vi "Periodic Tasks.vi"(8 "error in (no error)":errorcluster) -> ()   [LabVIEW 2012]
doc: "This VI runs in parallel to other tasks. It can contain as many user-defined periodic loops as you need. These can carry out PID or other sorts of timed response."
uses:
  <vilib>/Rock Robotics/SystemInterfaces/Utilities/FPGA_UtilitiesLED Source.ctl
  <vilib>/Rock Robotics/SystemInterfaces/Utilities/FPGA_UtilitiesLED State.ctl
  <vilib>/Rock Robotics/WPI/Solenoid/WPI_SolenoidValue.ctl
  <vilib>/Rock Robotics/WPI/Compressor/WPI_CompressorGetSetRefNum.vi
  System Set Points and States.vi
  <vilib>/Rock Robotics/WPI/Solenoid/WPI_SolenoidSetEnum.vi
  Robot Global Data.vi
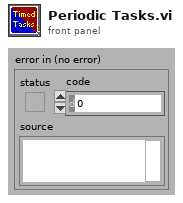
[diagram p1: front panel]
types:
  T1 = typedef "FPGA_UtilitiesLED State.ctl" = enum16{"Off", "On", "Toggle"}
  T2 = typedef "FPGA_UtilitiesLED Source.ctl" = enum16{"User LED", "FPGA LED"}
  T3 = typedef "WPI_SolenoidValue.ctl" = enum16{"Off", "On", "Forward", "Reverse"}
  T4 = typedef "WPI_SolenoidDevRef.ctl" = cluster{"DevStatus":errorcluster, "Solenoid Module":T5, "Forward Solenoid Channel":T6, "Reverse Solenoid Channel":T6}
  T5 = typedef "FPGA_TypedefSolenoidModule.ctl" = enum16{"Solenoid Module 1", "Solenoid Module 2"}
  T6 = typedef "WPI_SolenoidChannel.ctl" = enum8{"Solenoid 1", "Solenoid 2", "Solenoid 3", "Solenoid 4", "Solenoid 5", "Solenoid 6", "Solenoid 7", "Solenoid 8", "Invalid"}
  T7 = typedef "WPI_MotorControlDeviceRef.ctl" = cluster{"DeviceStatus":errorcluster, "Type":enum16{"PWM", "CAN"}, "PWM":cluster{"Digital Module":T8, "PWM Channel":T9, "DeadBand":T10}, "CAN":cluster{"Device Number":u8, "Control Mode":T11, "Semaphore":T12, "Max Vout":dbl}, "Invert":bool, "TransformRef":T13, "InvTransformRef":T13}
  T8 = typedef "FPGA_TypedefDigitalModule.ctl" = enum16{"Digital Module 1", "Digital Module 2"}
  T9 = typedef "FPGA_DIOPWMChannel.ctl" = enum8{"PWM 1", "PWM 2", "PWM 3", "PWM 4", "PWM 5", "PWM 6", "PWM 7", "PWM 8", "PWM 9", "PWM 10", "Invalid"}
  T10 = typedef "WPI_PWMDeadband.ctl" = cluster{"Name":string, "maxPositivePwm":i32, "minPositivePwm":i32, "centerPwm":i32, "maxNegativePwm":i32, "minNegativePwm":i32, "angularRange":u16}
  T11 = typedef "WPI_CANJaguar_ControlMode.ctl" = enum8{"Percent VBus", "Current", "Speed", "Position", "Voltage"}
  T12 = typedef "Semaphore RefNum" = refnum<k1>
  T13 = typedef "WPI_PWMTransform_ConPane.ctl" = refnum<vi>
  T14 = typedef "WPI_CompressorDevRef.ctl" = cluster{"DevStatus":errorcluster, "DigitalInputDevRef":T15, "RelayDevRef":T17}
  T15 = typedef "WPI_DigitalInputDevRef.ctl" = cluster{"DevStatus":errorcluster, "DIO Channel":T16, "Digital Module":T8}
  T16 = typedef "FPGA_DIOChannel.ctl" = enum8{"DIO 1", "DIO 2", "DIO 3", "DIO 4", "DIO 5", "DIO 6", "DIO 7", "DIO 8", "DIO 9", "DIO 10", "DIO 11", "DIO 12", "DIO 13", "DIO 14", "Invalid"}
  T17 = typedef "WPI_RelayDevRef.ctl" = cluster{"DevStatus":errorcluster, "Relay Channel":T18, "Digital Module":T8, "Relay Direction":T19}
  T18 = typedef "FPGA_DIORelayChannel.ctl" = enum8{"Relay 1", "Relay 2", "Relay 3", "Relay 4", "Relay 5", "Relay 6", "Relay 7", "Relay 8", "Invalid"}
  T19 = typedef "WPI_RelayDirection.ctl" = enum16{"Both directions", "Forward only", "Reverse only"}
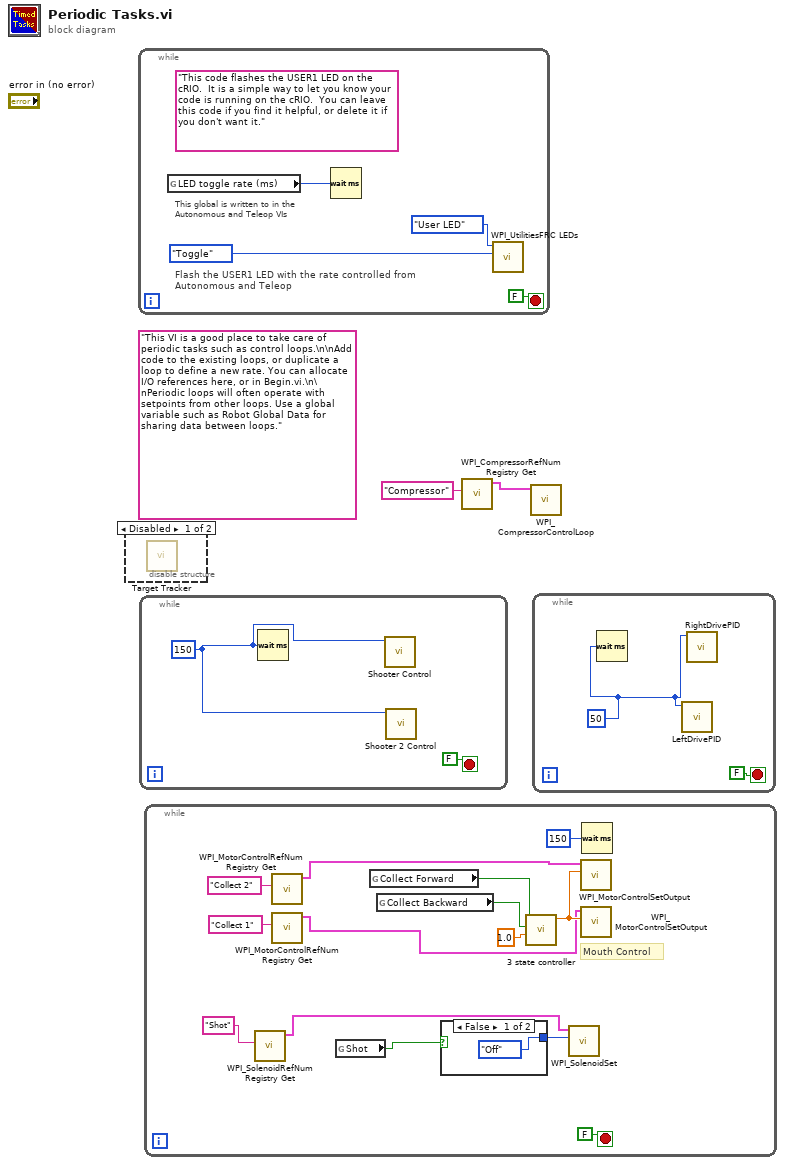
[diagram p0: block diagram]
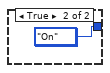
[diagram p2: hidden frame]
diagram:
  (unwired) "This VI is a good place to take care of periodic tasks such as control loops.\n\nAdd code to the existing loops, or duplicate a loop to define a new rate. You can allocate I/O references here, or in Begin.vi.\n\nPeriodic loops will often operate with setpoints from other loops. Use a global variable such as Robot Global Data for sharing data between loops."
  n1 = disable-structure shown="Disabled" {
    frame Disabled {
      n2 = call "Target Tracker.vi"() -> ()  [unwired: 12 in]
    }
    frame Enabled {
    }
  }
  n3 = while {
    stop <- FALSE stop-if-true
    (unwired) "This code flashes the USER1 LED on the cRIO.  It is a simple way to let you know your code is running on the cRIO.  You can leave this code if you find it helpful, or delete it if you don't want it."
    # "This global is written to in the Autonomous and Teleop VIs"
    # "Flash the USER1 LED with the rate controlled from Autonomous and Teleop"
    n4 = global read "Robot Global Data.vi" "LED toggle rate (ms)"() -> (w3:u32)
    n5 = Wait (ms)(milliseconds to wait=w3) -> ()  [unwired: 1 out]
    n6 = call <vilib>:"WPI_UtilitiesFRC LEDs.vi"("State"=FPGA_UtilitiesLED_State."Toggle", "LED Type"=FPGA_UtilitiesLED_Source."User LED") -> ()  [unwired: 1 in, 9 out]
  }
  n7 = while {
    stop <- FALSE stop-if-true
    w7 = u32 150
    n8 = Wait (ms)(milliseconds to wait=w7) -> ()  [unwired: 1 out]
    n9 = call "Shooter Control.vi"("Time Delay Milli"=w7) -> ()  [unwired: 11 in]
    n10 = call "Shooter 2 Control.vi"("Time Delay Milli"=w7) -> ()  [unwired: 11 in]
  }
  n11 = while {
    stop <- FALSE stop-if-true
    # "Mouth Control"
    n12 = call <vilib>:"WPI_SolenoidRefNum Registry Get.vi"("refnum name"="Shot") -> ("SolenoidDevRef"=w11:T4)  [unwired: 9 in, 1 out]
    n13 = call <vilib>:"WPI_MotorControlRefNum Registry Get.vi"("refnum name"="Collect 2") -> ("MotorControlDevRef"=w15:T7)  [unwired: 9 in, 1 out]
    n14 = call <vilib>:"WPI_MotorControlRefNum Registry Get.vi"("refnum name"="Collect 1") -> ("MotorControlDevRef"=w18:T7)  [unwired: 9 in, 1 out]
    n15 = global read "System Set Points and States.vi" "Shot"() -> (w10:bool)
    n16 = global read "System Set Points and States.vi" "Collect Forward"() -> (w14:bool)
    n17 = global read "System Set Points and States.vi" "Collect Backward"() -> (w13:bool)
    n18 = case shown="False" w10 {
      tunnel: [WPI_SolenoidValue."Off" ("Value") WPI_SolenoidValue."On" ("Value")] -> w12
      frame False {
      }
      frame True {
        (unwired) WPI_SolenoidValue."On" ("Value")
      }
    }
    n19 = call "3 state controller.vi"("Power"=1.0, "Backward"=w13, "Forward"=w14) -> ("Numeric"=w19:dbl)  [unwired: 8 in]
    n20 = call-poly <vilib>:"WPI_SolenoidSet.vi"("Value"=w12, "SolenoidDevRef"=w11) -> ()  [unwired: 8 in, 2 out]
    n21 = call <vilib>:"WPI_MotorControlSetOutput.vi"("Output"=w19, "MotorControlDevRef"=w15) -> ()  [unwired: 7 in, 3 out]
    n22 = call <vilib>:"WPI_MotorControlSetOutput.vi"("Output"=w19, "MotorControlDevRef"=w18) -> ()  [unwired: 7 in, 3 out]
    n23 = Wait (ms)(milliseconds to wait=u32 150) -> ()  [unwired: 1 out]
  }
  n24 = call <vilib>:"WPI_CompressorRefNum Registry Get.vi"("refnum name"="Compressor") -> ("CompressorDevRef"=w2:T14)  [unwired: 9 in, 1 out]
  n25 = call <vilib>:"WPI_CompressorControlLoop.vi"("CompressorDevRef"=w2) -> ()  [unwired: 11 in]
  n26 = while {
    stop <- FALSE stop-if-true
    w26 = u32 50
    n27 = Wait (ms)(milliseconds to wait=w26) -> ()  [unwired: 1 out]
    n28 = call "LeftDrivePID.vi"("Time Delay Milli"=w26) -> ()  [unwired: 11 in]
    n29 = call "RightDrivePID.vi"("Time Delay Milli"=w26) -> ()  [unwired: 11 in]
  }
